vi "Setup.vi"(11 "Hello World Queue in":refnum<class "Hello World Queue.lvclass">) -> (3 "Hello World Queue out":refnum<class "Hello World Queue.lvclass">)   [LabVIEW 2021, in "Hello World Queue.lvlib" / "Hello World Queue.lvclass"]
uses:
  Hello World Queue.lvclass
  Hello World Event/Hello World Event/Hello World Event.lvclass
  C:/git/jettl/src/jettl/jettl/Event jettl/Event jettl.lvclass
  Hello World Queue.lvclass/Hello World Queue.ctl
  jettl/Queue jettl/Queue jettl.lvclass
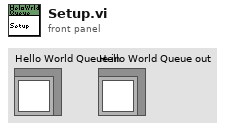
[diagram p1: front panel]
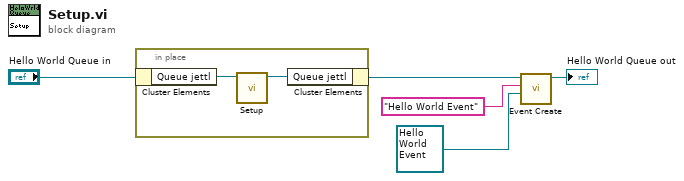
[diagram p0: block diagram]
diagram:
  n1 = in-place {
    n2 = in-place-cluster #1("Hello World Queue in") -> ("Queue jettl"=w7:refnum<class "Queue jettl.lvclass">)
    n3 = call-dynamic "Setup.vi"("Setup in"=w7) -> ("Setup out"=w6:refnum<class "Queue jettl.lvclass">)  [unwired: 10 in]
    n4 = in-place-cluster #1("Queue jettl"=w6) -> (w4:refnum<class "Hello World Queue.lvclass">)
  }
  n5 = call-dynamic "Event Create.vi"("Event jettl"=refnum<class "Hello World Event.lvclass"> refnum ("Hello World Event.lvlib:Hello World Event.lvclass"), "Alias"="Hello World Event", "Hello World Queue in"=w4) -> ("Hello World Queue out"=→"Hello World Queue out":refnum<class "Hello World Queue.lvclass">)  [unwired: 8 in]
